vi "Connect8742.vi"(8 "error in (no error)":errorcluster, 11 "Picomotor8742Comm in":refnum<class "PicoMotor8742Comm.lvclass">) -> (0 "error out":errorcluster, 3 "Picomotor8742Comm out":refnum<class "PicoMotor8742Comm.lvclass">)   [LabVIEW 2020, in "PicoMotor8742Comm.lvclass"]
uses:
  PicoMotor8742Comm.lvclass
  PicoMotor8742Comm.lvclass/PicoMotor8742Comm.ctl
  ASCIICommClass.lvclass
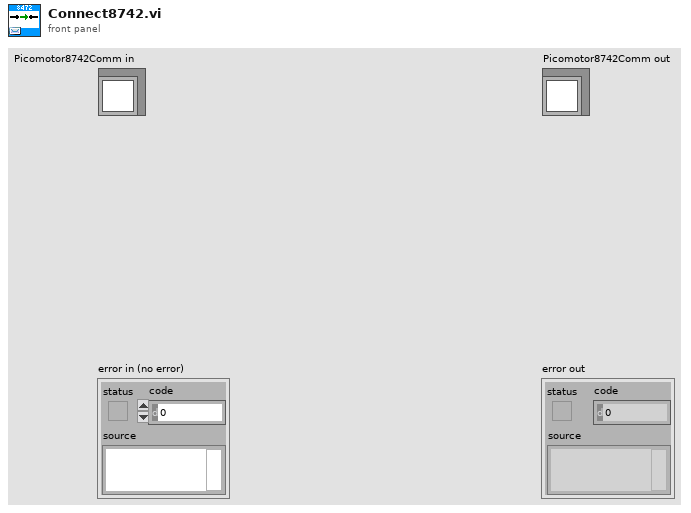
[diagram p1: front panel]
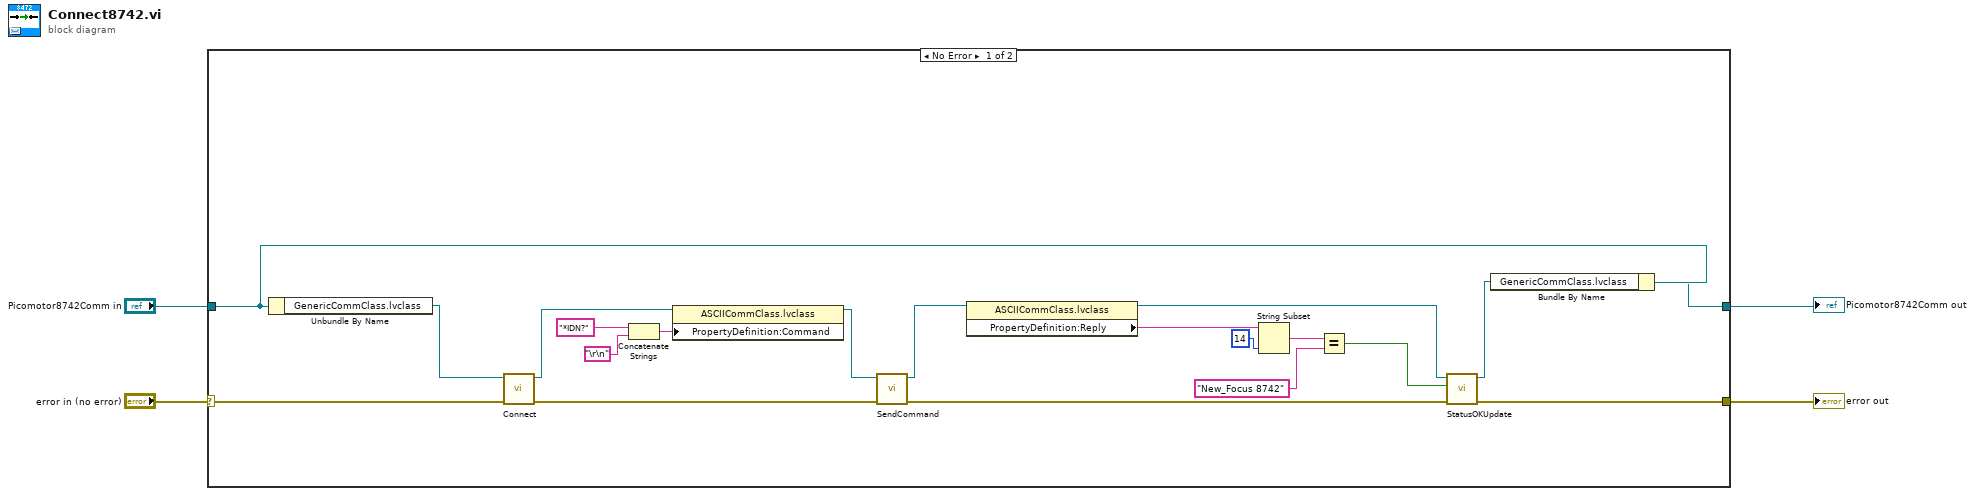
[diagram p0: block diagram]
diagram:
  n1 = case shown="No Error" "error in (no error)" {
    selector: "error in (no error)" -> [w20 w25]
    tunnel: [w18 w25] -> w3
    tunnel: "Picomotor8742Comm in" -> [w14 w24]
    tunnel: [w13 w24] -> w1
    frame No Error {
      n2 = Unbundle By Name(w14) -> ("GenericCommClass.lvclass"=w21:refnum<class "ASCIICommClass.lvclass">)
      n3 = call-dynamic "Connect.vi"("error in (no error)"=w20, "GenericCommClass in"=w21) -> ("error out"=w19:errorcluster, "GenericCommClass out"=w7:refnum<class "ASCIICommClass.lvclass">)  [unwired: 8 in]
      n4 = Concatenate Strings("*IDN?" ("Data.Command"), "\r\n") -> (w6:string)
      n5 = property class="ASCIICommClass.lvclass"(reference=w7, "PropertyDefinition:Command"=w6) -> (reference out=w5:refnum<class "ASCIICommClass.lvclass">)  [unwired: 1 in, 1 out]
      n6 = call-dynamic "SendCommand.vi"("error in (no error)"=w19, "GenericCommClass in"=w5) -> ("error out"=w18:errorcluster, "GenericCommClass out"=w17:refnum<class "ASCIICommClass.lvclass">)  [unwired: 8 in]
      n7 = property class="ASCIICommClass.lvclass"(reference=w17) -> (reference out=w15:refnum<class "ASCIICommClass.lvclass">, "PropertyDefinition:Reply"=w16:string)  [unwired: 1 in, 1 out]
      n8 = String Subset(string=w16, length (rest)=14 ("length (rest)")) -> (substring=w10:string)  [unwired: 1 in]
      n9 = Equal?(x=w10, y="New_Focus 8742" ("x")) -> (x = y?=w22:bool)
      n10 = call-dynamic "StatusOKUpdate.vi"("error in (no error)"=w18, "OkIn"=w22, "Picomotor8742Comm in"=w15) -> ("Picomotor8742Comm out"=w12:refnum<class "ASCIICommClass.lvclass">)  [unwired: 7 in, 1 out]
      n11 = Bundle By Name(cluster=w14, "GenericCommClass.lvclass"=w12) -> (w13:refnum<class "PicoMotor8742Comm.lvclass">)
    }
    frame Error {
    }
  }
  "error out" <- w3
  "Picomotor8742Comm out" <- w1
